vi "HFRR ADV v07.vi"() -> ()   [LabVIEW 2025] (continued)
            n4061 = call <vilib>:"MB Serial Init.vi"("Timeout"=u32 100, "Flow Control"=w5692, "Mode"=w5693, "error in (no error)"=w5690, "Parity"=w5691, "Baud Rate"=u32 9600, "VISA resource name"="Lubrication System COM Port :") -> ("error out"=w5679:errorcluster, "VISA resource name out"=w5687:refnum<visa-resource-name>)  [unwired: 3 in]
            n4062 = local write "set temp old"(0.0 ("set temp old")) -> ()
            n4063 = Unbundle(w5679) -> ("status"=w5678:bool)  [unwired: 2 out]
            n4064 = case shown="True" w5678 {
              selector: w5678 -> [_ w5695]
              frame False {
              }
              frame True {
                n4065 = local write "TK4 status"(w5695) -> ()
              }
            }
          }
        }
        n4066 = local read "Quit"() -> (w5599:bool)
      }
      n4067 = VISA Close(VISA resource name=w5595, error in (no error)=w5596) -> (error out=w5594:errorcluster)
      n4068 = call <vilib>:"Clear Errors.vi"("error in (no error)"=w5594) -> ()  [unwired: 5 in, 2 out]
    }
    frame Enabled {
    }
  }
  "file count" <- 0 ("file count")
